vi "EnQmsg.vi"(6 "timeout in ms (-1)":i32, 7 "priority?":bool, 8 "error in (no error)":errorcluster, 9 "payload":variant, 10 "message":string, 11 "EnQin":T1) -> (0 "error out":errorcluster, 3 "EnQout":refnum<queue>, 4 "timed out?":bool)   [LabVIEW 2021]
uses:
  EnQcmd.ctl
  EnQref.ctl
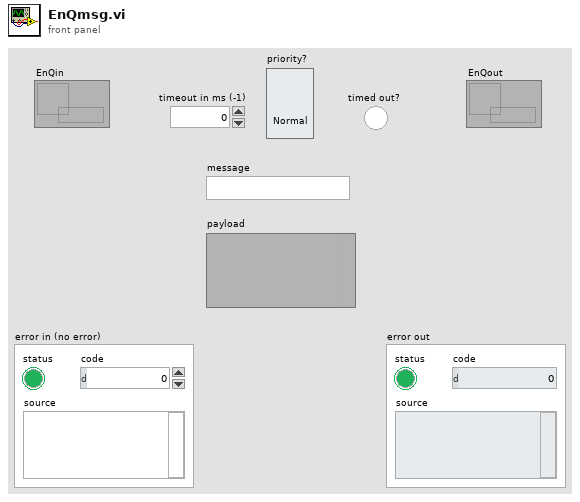
[diagram p1: front panel]
types:
  T1 = typedef "EnQref.ctl" = refnum<queue>
  T2 = typedef "EnQcmd.ctl" = cluster{"message":string, "payload":variant}
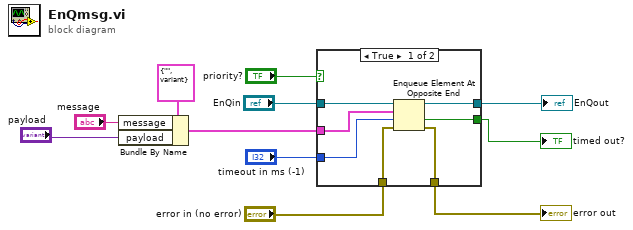
[diagram p0: block diagram]
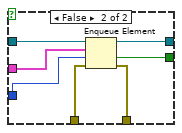
[diagram p2: hidden frame]
diagram:
  n1 = Bundle By Name(cluster=T2 {"message"="", "payload"=variant} ("command"), "message"="message", "payload"="payload") -> (w3:T2)
  n2 = case shown="True" "priority?" {
    tunnel: "EnQin" -> [w18 w25]
    tunnel: [w17 w24] -> w2
    tunnel: "error in (no error)" -> [w16 w23]
    tunnel: [w15 w22] -> w10
    tunnel: [w14 w21] -> w9
    tunnel: "timeout in ms (-1)" -> [w13 w20]
    tunnel: w3 -> [w12 w19]
    frame True {
      n3 = Enqueue Element At Opposite End(queue=w18, element=w12, timeout in ms (-1)=w13, error in (no error)=w16) -> (queue out=w17:T1, timed out?=w14:bool, error out=w15:errorcluster)
    }
    frame False {
      n4 = Enqueue Element(queue=w25, element=w19, timeout in ms (-1)=w20, error in (no error)=w23) -> (queue out=w24:T1, timed out?=w21:bool, error out=w22:errorcluster)
    }
  }
  "error out" <- w10
  "timed out?" <- w9
  "EnQout" <- w2
